vi "coordinated led control panel with logging and directory support.vi"() -> ()   [LabVIEW 2013]
uses:
  Image Aquisition - Labview/Image Recorder/experiment state global.vi
panel:
  in  "LOGARITHMIC output":bool
  in  "lednumber":u8=1 min=1 max=2
  in  "enable output 2":bool
  out "directory2 contents":string[](array[string])
  in  "led2 destination directory":string
  in  "led2 input directory":path
  in  "file name 2":u16(ring) items=["20140619/1523/2/12.bin", "20140619/1523/2/128.bin", "20140619/1523/2/255.bin", "20140619/1523/2/5.bin"]
  in  "enable output 1":bool
  in  "output enabled":bool
  in  "stimulus2 value":u8
  out "transfer in progress":bool
  out "directory1 contents":string[](array[string])
  in  "transfer files":bool
  in  "led1 destination directory":string
  in  "led1 input directory":path
  in  "stimulus1 value":u8
  in  "clear history":bool
  out "info":T1
  out "history":string
  in  "num bytes per frame":u32=8
  in  "file name 1":u16(ring) items=["20140623/1248/1/23june1.bin", "20140623/1248/1/23june10.bin", "20140623/1248/1/23june2.bin", "20140623/1248/1/23june3.bin", "20140623/1248/1/23june4.bin", "20140623/1248/1/23june5.bin", "20140623/1248/1/23june6.bin", "20140623/1248/1/23june7.bin", "20140623/1248/1/23june8.bin", "20140623/1248/1/23june9.bin"]
  out "byte data":u8[](array[numeric])
  in  "update time (ms)":i32=50
  out "serial set up OK?":bool
  out "error out":errorcluster
  in  "stop":bool
  in  "Command":T2(ring)
  in  "Execute Command":bool
  in  "Teensy Serial Port Name":refnum<visa-resource-name>="COM3"
  # "note: set stimulus state does not care if output is enabled/disabled"
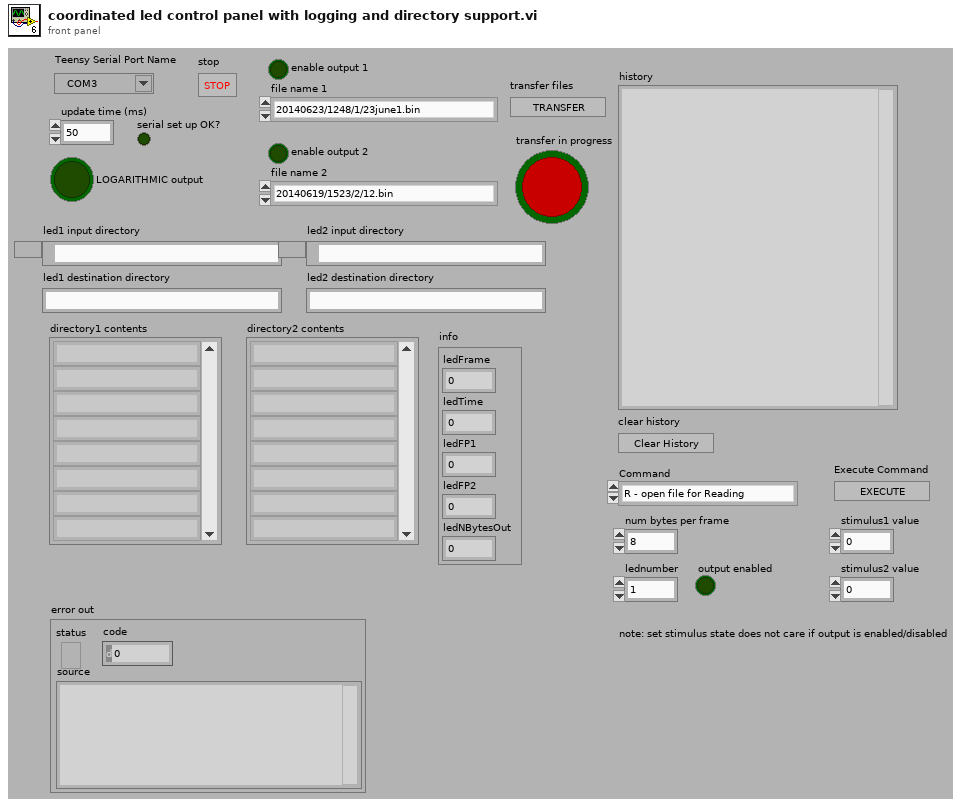
[diagram p1: front panel]
types:
  T1 = cluster{"ledFrame":i32, "ledTime":i32, "ledFP1":i32, "ledFP2":i32, "ledNBytesOut":i32}
  T2 = enum16{"R - open file for Reading", "W - open file for Writing", "S - send bytes", "F - fetch bytes", "B - begin experiment", "E - end experiment", "N - set number of bits per frame", "I - get info", "Q - Quiet (only error msgs)", "L - Loud (acknowledge all)", "T - set stimulus state", "Y - ready to start experiment", "H - useless Help message", "C - Close file", "O - enable/disable output", "G - set logarithmic output"}
  T3 = enum16{"R - open file for Reading", "W - open file for Writing", "S - send bytes", "F - fetch bytes", "B - begin experiment", "E - end experiment", "N - set number of bits per frame", "I - get info", "Q - Quiet (only error msgs)", "L - Loud (acknowledge all)", "T - set stimulus state", "Y - ready to start experiment", "H - useless Help message", "C - Close file", "O - enable/disable output"}
  T4 = cluster{"experiment started":bool, "experiment ended":bool, "experiment start time":u32}
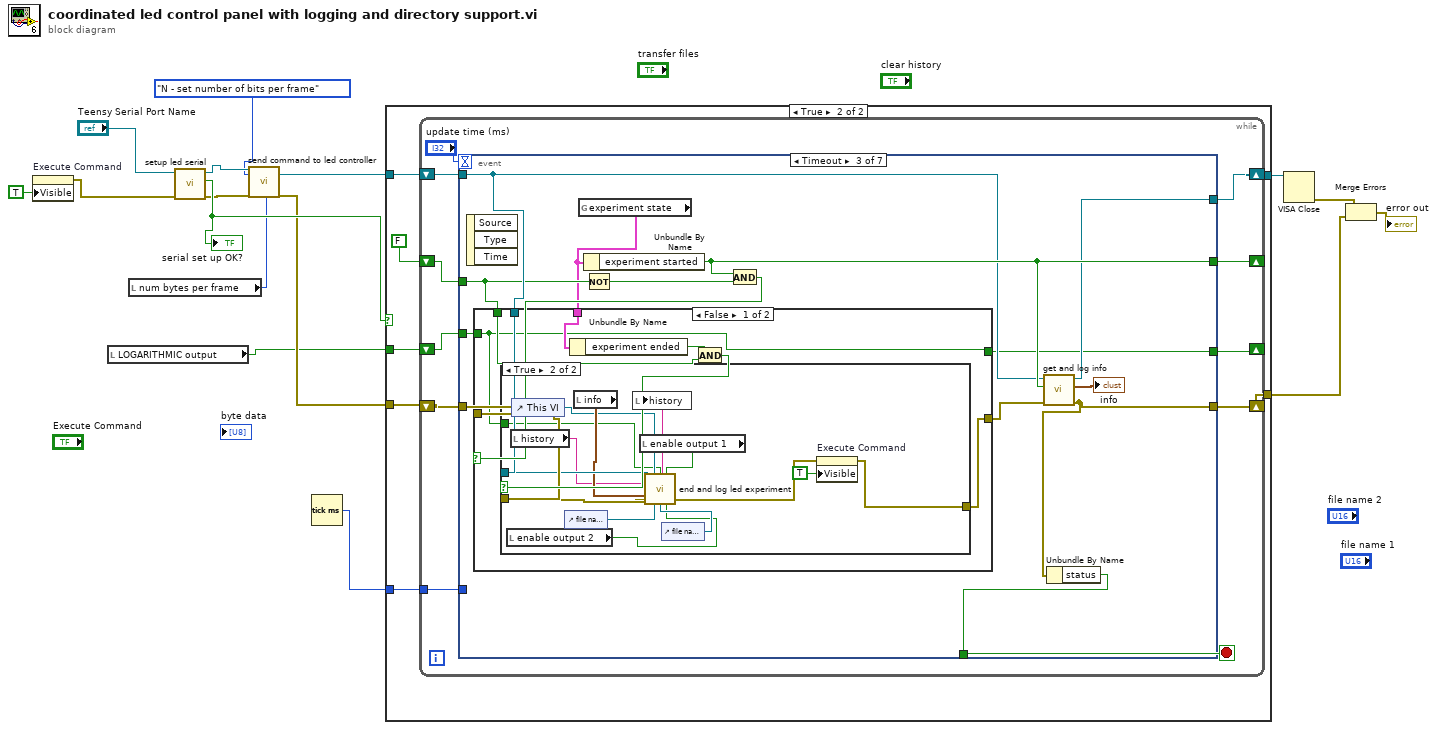
[diagram p0: block diagram]
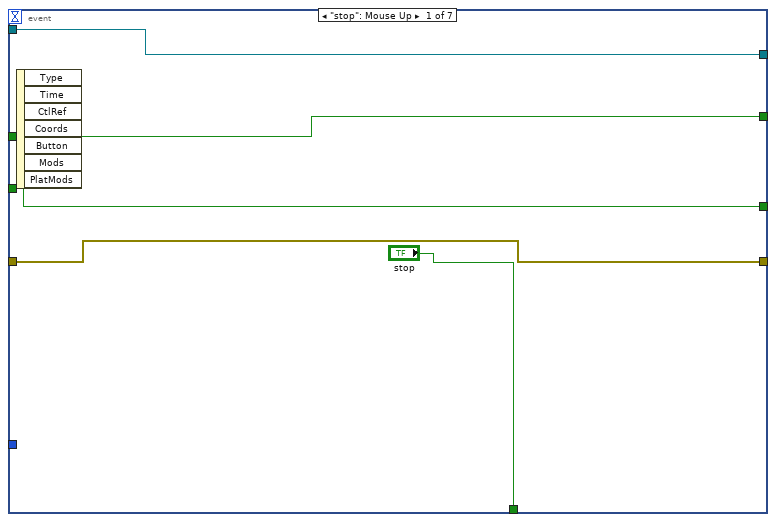
[diagram p3: hidden frame]
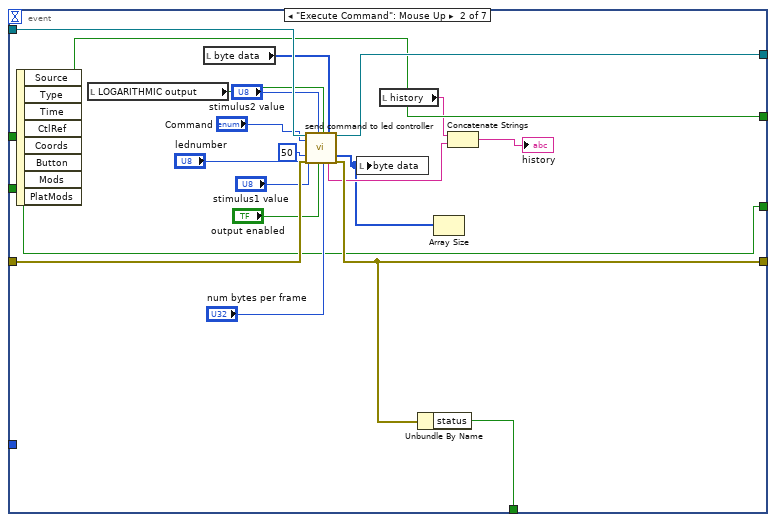
[diagram p4: hidden frame]
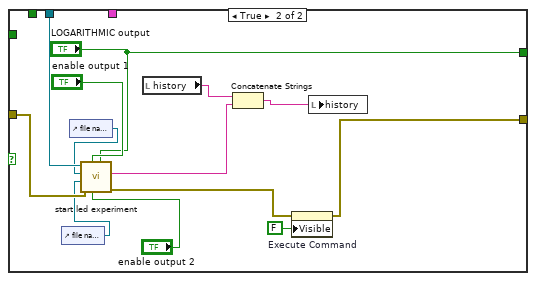
[diagram p6: hidden frame]
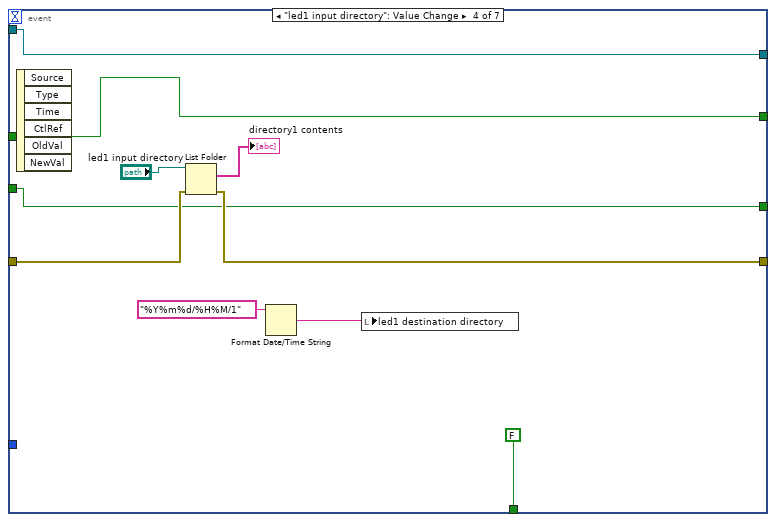
[diagram p7: hidden frame]
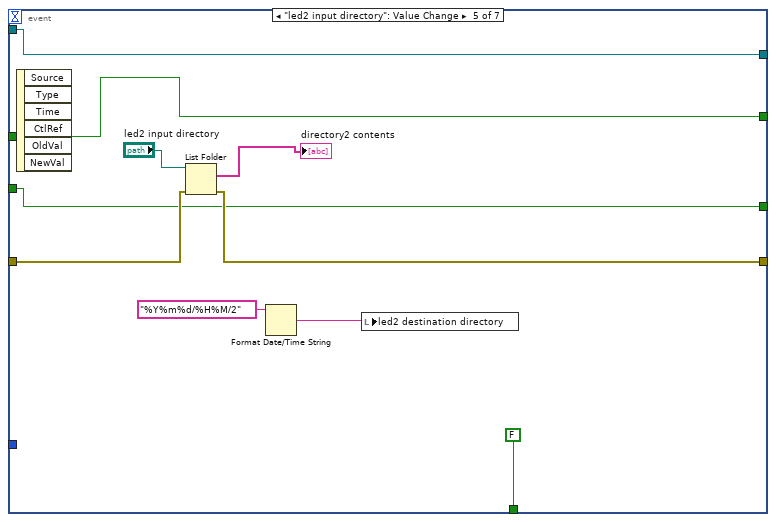
[diagram p8: hidden frame]
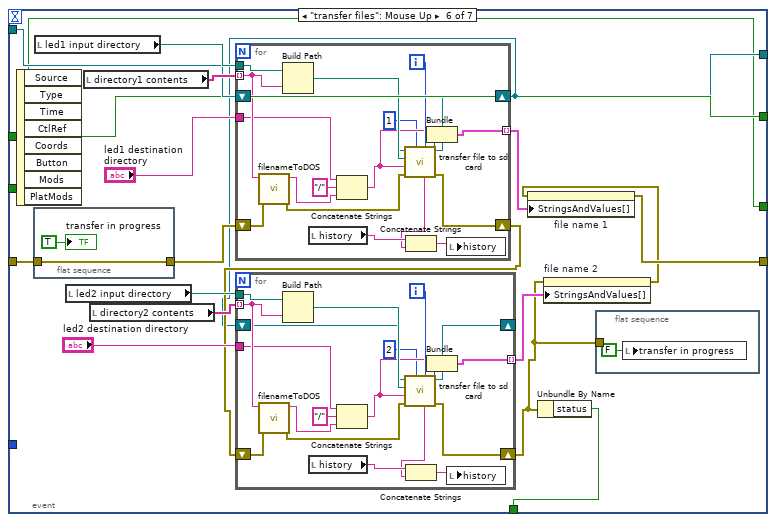
[diagram p9: hidden frame]
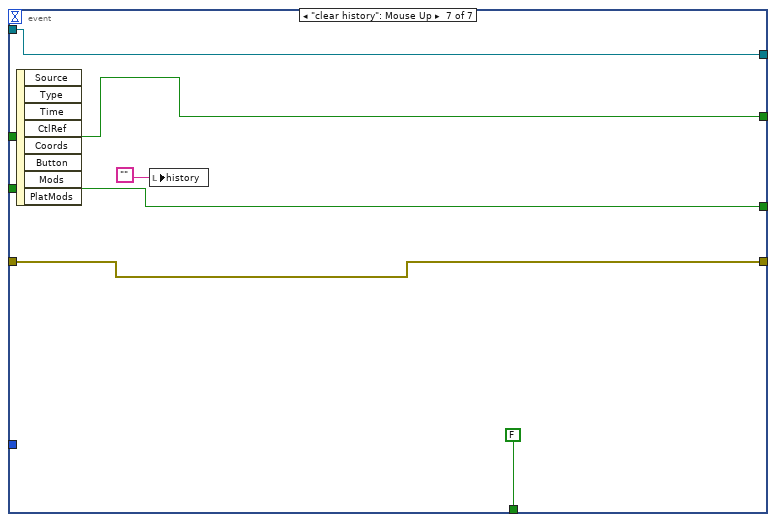
[diagram p10: hidden frame]
diagram:
  n1 = property on="Execute Command" class="Bool (strict)"("Visible"=TRUE) -> (error out=w2:errorcluster)  [unwired: 2 in, 1 out]
  n2 = local read "LOGARITHMIC output"() -> (w3:bool)
  n3 = local read "num bytes per frame"() -> (w5:u32)
  n4 = call "setup led serial.vi"("error in (no error)"=w2, "Teensy Serial Port"="Teensy Serial Port Name") -> ("error out"=w9:errorcluster, "OK"=w11:bool, "Teensy Serial Port"=w7:refnum<visa-resource-name>)  [unwired: 7 in]
  "serial set up OK?" <- w11
  n5 = call "send command to led controller.vi"("Teensy Serial Port"=w7, "Command"=T3."N - set number of bits per frame", "error in"=w9, "num bits per frame"=w5) -> ("teensy serial port out"=w6:refnum<visa-resource-name>, "error out"=w8:errorcluster)  [unwired: 10 in, 4 out]
  n6 = Tick Count (ms)() -> (millisecond timer value=w10:u32)
  n7 = case shown="True" w11 {
    tunnel: [w18 w25] -> w15
    tunnel: [w17 w24] -> w13
    tunnel: w8 -> [w17 w23]
    tunnel: w6 -> [w18 w22]
    tunnel: w10 -> [_ w20]
    tunnel: w3 -> [_ w19]
    frame False {
    }
    frame True {
      n8 = while {
        shift-right: [w35] -> w24
        shift-left: w23 -> [w36]
        shift-right: [w32] -> w25
        shift-left: w22 -> [w34]
        shift-right: [w30] -> _
        shift-left: FALSE ("experiment started") -> [w29]
        tunnel: w20 -> [w28]
        shift-right: [w27] -> _
        shift-left: w19 -> [w26]
        stop <- w33 stop-if-true
        n9 = event shown="[2] Timeout" {
          selector: _ -> [_ _ _ _ _ _ _]
          dyn-events: _ -> [_ _ _ _ _ _ _]
          timeout: "update time (ms)" -> [_ _ _ _ _ _ _]
          tunnel: w36 -> [w40 w61 w74 w117 w128 w150 w194]
          tunnel: [w40 w56 w70 w115 w127 w143 w194] -> w35
          tunnel: w34 -> [w39 w60 w66 w120 w130 w146 w193]
          tunnel: [w39 w59 w68 w120 w130 w133 w193] -> w32
          tunnel: ["stop" w55 w72 FALSE ("status") FALSE ("status") w145 FALSE ("status")] -> w33
          tunnel: [w38 w57 w69 w119 w129 w144 w192] -> w30
          tunnel: w29 -> [w38 w57 w65 w119 w129 w144 w192]
          tunnel: w28 -> [_ _ _ _ _ _ _]
          tunnel: [w37 w42 w63 w112 w122 w132 w190] -> w27
          tunnel: w26 -> [w37 w42 w62 w112 w122 w132 w190]
          event "stop": Mouse Up {
            n10 = event-data() -> ()  [unwired: 1 in, 7 out]
          }
          event "Execute Command": Mouse Up {
            n11 = event-data() -> ()  [unwired: 1 in, 8 out]
            n12 = local read "LOGARITHMIC output"() -> (w43:bool)
            n13 = local read "byte data"() -> (w53:u8[])
            n14 = call "send command to led controller.vi"("Teensy Serial Port"=w60, "Command"="Command", "lednumber"="lednumber", "stimulus1 value"="stimulus1 value", "milliseconds to wait between write and read"=u32 50, "error in"=w61, "stimulus2 value"="stimulus2 value", "output enabled"="output enabled", "logarithmic output?"=w43, "num bits per frame"="num bytes per frame", "bytes to send"=w53) -> ("command and response with time"=w50:string, "teensy serial port out"=w59:refnum<visa-resource-name>, "bytes read"=w47:u8[], "error out"=w56:errorcluster)  [unwired: 3 in, 2 out]
            n15 = local write "byte data"(w47) -> ()
            n16 = local read "history"() -> (w51:string)
            n17 = Unbundle By Name(w56) -> ("status"=w55:bool)
            n18 = Array Size(array=w47) -> ()  [unwired: 1 out]
            n19 = Concatenate Strings(w51, w50) -> (→"history":string)
          }
          event Timeout {
            n20 = event-data() -> ()  [unwired: 1 in, 3 out]
            n21 = global read "experiment state global.vi" "experiment state"() -> (w64:T4)
            n22 = Unbundle By Name(w64) -> ("experiment started"=w69:bool)
            n23 = Not(x=w65) -> (.not. x?=w75:bool)
            n24 = And(x=w69, y=w75) -> (x .and. y?=w73:bool)
            n25 = case shown="False" w73 {
              tunnel: w74 -> [w78 w111]
              tunnel: [w77 w99] -> w71
              tunnel: w66 -> [w79 w110]
              tunnel: w65 -> [w81 _]
              tunnel: w64 -> [w83 _]
              tunnel: [w76 "LOGARITHMIC output"] -> w63
              tunnel: w62 -> [w76 _]
              frame False {
                n26 = Unbundle By Name(w83) -> ("experiment ended"=w82:bool)
                n27 = And(x=w82, y=w81) -> (x .and. y?=w80:bool)
                n28 = case shown="True" w80 {
                  tunnel: w79 -> [_ w97]
                  tunnel: w78 -> [w84 w98]
                  tunnel: [w84 w86] -> w77
                  tunnel: w76 -> [_ w88]
                  frame False {
                  }
                  frame True {
                    n29 = local read "enable output 2"() -> (w89:bool)
                    n30 = local read "history"() -> (w95:string)
                    n31 = control-ref of="This VI"() -> (w93:refnum<vi>)
                    n32 = control-ref of="file name 1"() -> (w92:refnum<vi>)
                    n33 = local read "info"() -> (w96:T1)
                    n34 = local read "enable output 1"() -> (w90:bool)
                    n35 = control-ref of="file name 2"() -> (w91:refnum<vi>)
                    n36 = call "end and log led experiment.vi"("Teensy Serial Port"=w97, "vi"=w93, "logarithmic output?"=w88, "output1 enabled"=w90, "history"=w95, "info"=w96, "error in"=w98, "file name 1 ref"=w92, "file name 2 ref"=w91, "output2 enabled"=w89) -> ("history out"=w94:string, "error out"=w87:errorcluster)  [unwired: 3 in, 1 out]
                    n37 = local write "history"(w94) -> ()
                    n38 = property on="Execute Command" class="Bool (strict)"(error in=w87, "Visible"=TRUE) -> (error out=w86:errorcluster)  [unwired: 1 in, 1 out]
                  }
                }
              }
              frame True {
                n39 = control-ref of="file name 2"() -> (w105:refnum<vi>)
                n40 = control-ref of="file name 1"() -> (w106:refnum<vi>)
                n41 = call "start led experiment.vi"("logarithmic output?"="LOGARITHMIC output", "output2 enabled"="enable output 2", "output1 enabled"="enable output 1", "error in"=w111, "file name 2 ref"=w105, "file name 1 ref"=w106, "Teensy Serial Port"=w110) -> ("error out"=w100:errorcluster, "commands and responses"=w108:string)  [unwired: 2 in, 1 out]
                n42 = local read "history"() -> (w109:string)
                n43 = Concatenate Strings(w109, w108) -> (w107:string)
                n44 = property on="Execute Command" class="Bool (strict)"(error in=w100, "Visible"=FALSE) -> (error out=w99:errorcluster)  [unwired: 1 in, 1 out]
                n45 = local write "history"(w107) -> ()
              }
            }
            n46 = call "get and log info.vi"("error in"=w71, "log data?"=w69, "Teensy Serial Port"=w66) -> ("error out"=w70:errorcluster, "info"=→"info":T1, "LADY GAGA v2 Serial Port out"=w68:refnum<visa-resource-name>)  [unwired: 6 in]
            n47 = Unbundle By Name(w70) -> ("status"=w72:bool)
          }
          event "led1 input directory": Value Change {
            n48 = event-data() -> ()  [unwired: 1 in, 6 out]
            n49 = List Folder(path="led1 input directory", error in=w117) -> (filenames=→"directory1 contents":string[], error out=w115:errorcluster)  [unwired: 2 in, 2 out]
            n50 = Format Date/Time String(time format string (%c)="%Y%m%d/%H%M/1") -> (date/time string=w113:string)  [unwired: 2 in]
            n51 = local write "led1 destination directory"(w113) -> ()
          }
          event "led2 input directory": Value Change {
            n52 = event-data() -> ()  [unwired: 1 in, 6 out]
            n53 = List Folder(path="led2 input directory", error in=w128) -> (filenames=→"directory2 contents":string[], error out=w127:errorcluster)  [unwired: 2 in, 2 out]
            n54 = Format Date/Time String(time format string (%c)="%Y%m%d/%H%M/2") -> (date/time string=w125:string)  [unwired: 2 in]
            n55 = local write "led2 destination directory"(w125) -> ()
          }
          event "transfer files": Mouse Up {
            n56 = event-data() -> ()  [unwired: 1 in, 8 out]
            n57 = flat-sequence {
              tunnel: w150 -> [w188]
              tunnel: [w188] -> w142
              frame #0 {
                "transfer in progress" <- TRUE ("transfer in progress")
              }
            }
            n58 = local read "led1 input directory"() -> (w149:path)
            n59 = local read "led2 input directory"() -> (w140:path)
            n60 = local read "directory1 contents"() -> (w148:string[])
            n61 = local read "directory2 contents"() -> (w138:string[])
            n62 = for {
              tunnel: w149 -> [w187]
              tunnel: w148 -> [w186] mode=indexing
              tunnel: "led1 destination directory" -> [w185]
              shift-right: [w180] -> w137
              shift-left: w142 -> [w175]
              shift-right: [w178] -> w133
              shift-left: w146 -> [w179]
              tunnel: [w177] -> w141 mode=indexing
              i -> [w176]
              n63 = call "filenameToDOS.vi"("error in (no error)"=w175, "file name"=w186) -> ("error out"=w182:errorcluster, "8.3 filename"=w183:string)  [unwired: 8 in]
              n64 = Build Path(base path=w187, name or relative path=w186) -> (appended path=w181:path)
              n65 = local read "history"() -> (w173:string)
              n66 = Concatenate Strings(w185, "/" ("string"), w183) -> (w174:string)
              n67 = call "transfer file to sd card.vi"("output number"=u8 1, "error in"=w182, "disk file name"=w174, "input file"=w181, "Teensy Serial Port"=w179) -> ("error out"=w180:errorcluster, "teensy serial port out"=w178:refnum<visa-resource-name>, "commands and responses"=w172:string)  [unwired: 4 in]
              n68 = Concatenate Strings(w173, w172) -> (w171:string)
              n69 = Bundle(w174, w176) -> (w177:cluster{string, i32})  [unwired: 1 in]
              n70 = local write "history"(w171) -> ()
            }
            n71 = for {
              tunnel: w140 -> [w168]
              tunnel: w138 -> [w167] mode=indexing
              tunnel: "led2 destination directory" -> [w166]
              shift-right: [w161] -> w135
              shift-left: w137 -> [w156]
              shift-right: [w159] -> _
              shift-left: w133 -> [w160]
              tunnel: [w158] -> w136 mode=indexing
              i -> [w157]
              n72 = call "filenameToDOS.vi"("error in (no error)"=w156, "file name"=w167) -> ("error out"=w163:errorcluster, "8.3 filename"=w164:string)  [unwired: 8 in]
              n73 = Build Path(base path=w168, name or relative path=w167) -> (appended path=w162:path)
              n74 = local read "history"() -> (w154:string)
              n75 = Concatenate Strings(w166, "/" ("string"), w164) -> (w155:string)
              n76 = call "transfer file to sd card.vi"("output number"=u8 2, "error in"=w163, "disk file name"=w155, "input file"=w162, "Teensy Serial Port"=w160) -> ("error out"=w161:errorcluster, "teensy serial port out"=w159:refnum<visa-resource-name>, "commands and responses"=w153:string)  [unwired: 4 in]
              n77 = Concatenate Strings(w154, w153) -> (w152:string)
              n78 = Bundle(w155, w157) -> (w158:cluster{string, i32})  [unwired: 1 in]
              n79 = local write "history"(w152) -> ()
            }
            n80 = Unbundle By Name(w135) -> ("status"=w145:bool)
            n81 = property on="file name 2" class="Ring (strict)"(error in=w135, "StringsAndValues[]"=w136) -> (error out=w134:errorcluster)  [unwired: 1 in, 1 out]
            n82 = property on="file name 1" class="Ring (strict)"(error in=w134, "StringsAndValues[]"=w141) -> (error out=w143:errorcluster)  [unwired: 1 in, 1 out]
            n83 = flat-sequence {
              tunnel: w135 -> [_]
              frame #0 {
                n84 = local write "transfer in progress"(FALSE ("transfer in progress")) -> ()
              }
            }
          }
          event "clear history": Mouse Up {
            n85 = event-data() -> ()  [unwired: 1 in, 8 out]
            n86 = local write "history"("") -> ()
          }
        }
      }
    }
  }
  n87 = VISA Close(VISA resource name=w15) -> (error out=w14:errorcluster)  [unwired: 1 in]
  n88 = Merge Errors(w14, w13) -> (→"error out":errorcluster)
